vi "1_Sorting_solution.vi"(11 "Input String":string) -> (3 "Sorted Array":dbl[](array[numeric]))   [LabVIEW 2014]
panel:
  # "Sort the Numbers in the Input String and list them \nin the Sorted Array\nsee the following example"
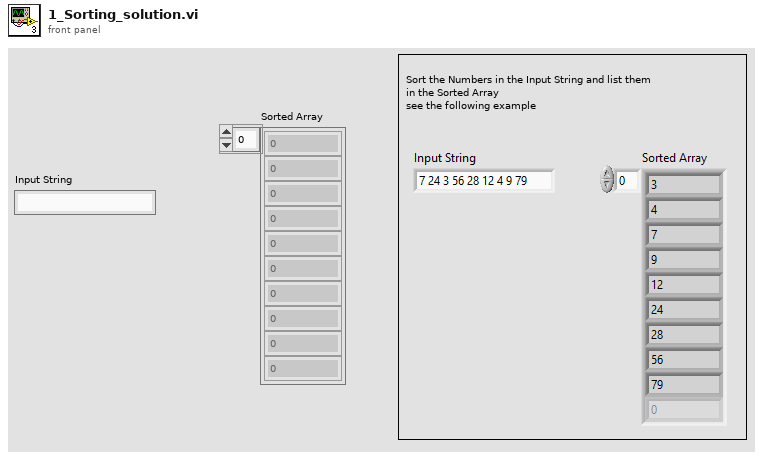
[diagram p1: front panel]
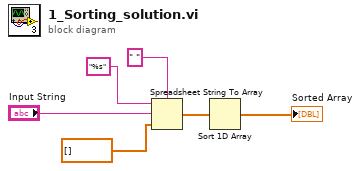
[diagram p0: block diagram]
diagram:
  n1 = Spreadsheet String To Array(delimiter (Tab)=" ", format string="%s", spreadsheet string="Input String", array type (2D Dbl)=dbl[] []) -> (array=w3:dbl[])
  n2 = Sort 1D Array(array=w3) -> (sorted array=→"Sorted Array":dbl[])
